vi "calculate last byte.vi"(10 "type":T1, 11 "byte in":i32) -> (3 "last byte":i32)   [LabVIEW 2013, in "Profibus Module runtime.lvclass"]
uses:
  Profibus Module runtime.lvclass
  <vilib>/NI/Tag Bus/tag/Data Type.ctl
  <vilib>/NI/Tag Bus/tag/tag descriptor.lvclass
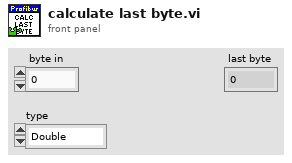
[diagram p1: front panel]
types:
  T1 = typedef "tag bus.lvlib/tag descriptor.lvclass/Data Type.ctl" = enum16{"Double", "Single", "I64", "I32", "I16", "I8", "U64", "U32", "U16", "U8", "Boolean", "String", "Array of Double", "Array of Single", "Array of I64", "Array of I32", "Array of I16", "Array of I8", "Array of U64", "Array of U32", "Array of U16", "Array of U8", "Array of Boolean", "Array of String"}
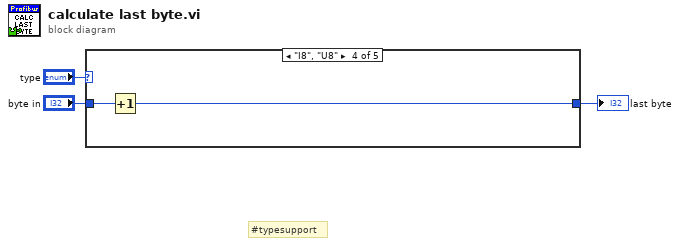
[diagram p0: block diagram]
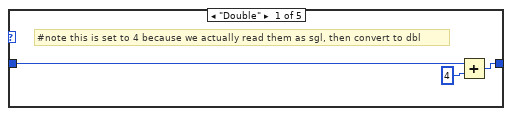
[diagram p2: hidden frame]
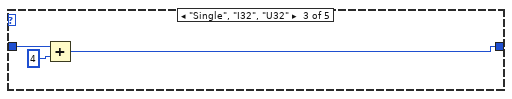
[diagram p4: hidden frame]
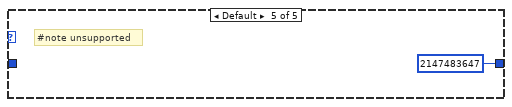
[diagram p5: hidden frame]
diagram:
  # "#typesupport"
  n1 = case shown="\"I8\", \"U8\"" "type" {
    tunnel: "byte in" -> [w4 w7 w10 w12 _]
    tunnel: [w5 w7 w8 w11 2147483647 ("byte in")] -> w1
    frame "Double" {
      # "#note this is set to 4 because we actually read them as sgl, then convert to dbl"
      n2 = Add(x=w4, y=4) -> (x+y=w5:i32)
    }
    frame "Boolean" {
    }
    frame "Single", "I32", "U32" {
      n3 = Add(x=w10, y=4) -> (x+y=w8:i32)
    }
    frame "I8", "U8" {
      n4 = Increment(x=w12) -> (x+1=w11:i32)
    }
    frame Default {
      # "#note unsupported"
    }
  }
  "last byte" <- w1
